vi "DtOLCreateTask.vi"   [LabVIEW 2016]
doc: "Creates one or more virtual channels, adds them to a task, and configures the task with the specified settings.\n\nThe instances of this polymorphic VI correspond to the type of subsystem on which the channel resides (analog input, analog output, digital input, digital output, counter/timer, or quadrature decoder), and the measurement or output operation to perform, such as voltage measurement, event counting, or rate generation."
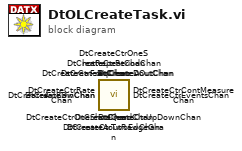
[diagram p0: block diagram]
diagram:
  n1 = call <userlib>:"DtCreateQuadChan.vi"() -> ()  [unwired: 14 in, 2 out]
  n2 = call <userlib>:"DtCreateDOutChan.vi"() -> ()  [unwired: 14 in, 2 out]
  n3 = call <userlib>:"DtCreateDinChan.vi"() -> ()  [unwired: 14 in, 2 out]
  n4 = call <userlib>:"DtCreateCtrContMeasureChan.vi"() -> ()  [unwired: 14 in, 2 out]
  n5 = call <userlib>:"DtCreateCtrTwoEdgeChan.vi"() -> ()  [unwired: 14 in, 2 out]
  n6 = call <userlib>:"DtCreateCtrPeriodChan.vi"() -> ()  [unwired: 14 in, 2 out]
  n7 = call <userlib>:"DtCreateCtrFreqChan.vi"() -> ()  [unwired: 14 in, 2 out]
  n8 = call <userlib>:"DtCreateCtrUpDownChan.vi"() -> ()  [unwired: 14 in, 2 out]
  n9 = call <userlib>:"DtCreateCtrRateChan.vi"() -> ()  [unwired: 13 in, 3 out]
  n10 = call <userlib>:"DtCreateCtrOneShotRepeatChan.vi"() -> ()  [unwired: 13 in, 3 out]
  n11 = call <userlib>:"DtCreateCtrOneShotChan.vi"() -> ()  [unwired: 13 in, 3 out]
  n12 = call <userlib>:"DtCreateCtrEventsChan.vi"() -> ()  [unwired: 14 in, 2 out]
  n13 = call <userlib>:"DtCreateAoutRawChan.vi"() -> ()  [unwired: 13 in, 3 out]
  n14 = call <userlib>:"DtCreateAoutChan.vi"() -> ()  [unwired: 13 in, 3 out]
  n15 = call <userlib>:"DtCreateAinRawChan.vi"() -> ()  [unwired: 13 in, 3 out]
  n16 = call <userlib>:"DtCreateAinChan.vi"() -> ()  [unwired: 13 in, 3 out]
